vi "finde2.vi"(8 "esize":i32=1, 9 "thresh":i32=1, 11 "inp array":i32[][](array[numeric])) -> (3 "locs":i32[][](array[numeric]))   [LabVIEW 2020]
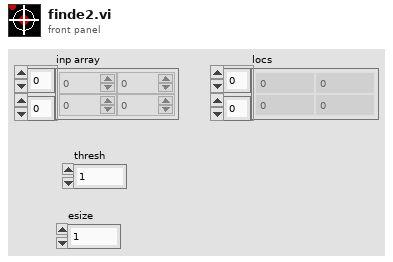
[diagram p1: front panel]
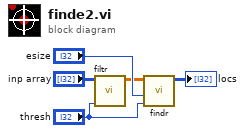
[diagram p0: block diagram]
diagram:
  n1 = call "filtr.vi"("lower threshold"="thresh", "input array"="inp array") -> ("output array"=w2:dbl[][])  [unwired: 9 in]
  n2 = call "findr.vi"("thresh"="thresh", "esize"="esize", "inp array"=w2) -> ("locs"=→"locs":i32[][])  [unwired: 8 in]
